vi "p72MomenInv.vi"(1 "Array 3":dbl[][](array[numeric])) -> (0 "appended array":dbl[](array[numeric]))   [LabVIEW 2013]
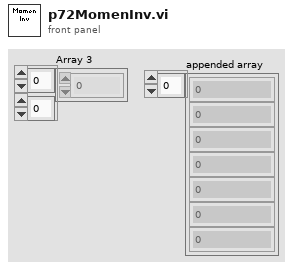
[diagram p1: front panel]
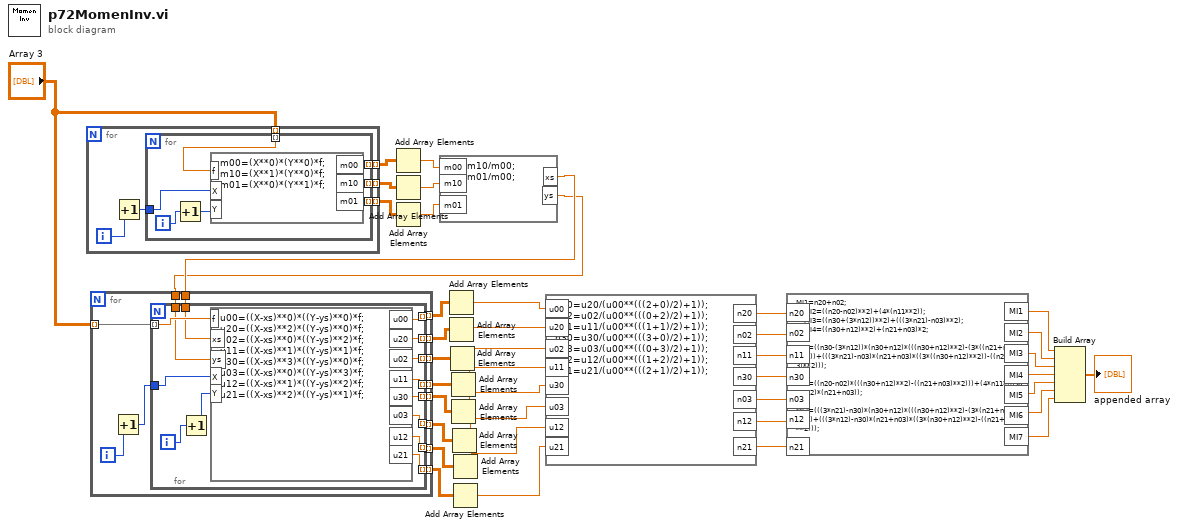
[diagram p0: block diagram]
diagram:
  n1 = for {
    tunnel: "Array 3" -> [w45] mode=indexing
    tunnel: [w43] -> w40 mode=indexing
    tunnel: [w42] -> w39 mode=indexing
    tunnel: [w41] -> w38 mode=indexing
    i -> [w46]
    n2 = Increment(x=w46) -> (x+1=w44:i32)
    n3 = for {
      tunnel: w45 -> [w53] mode=indexing
      tunnel: w44 -> [w52]
      tunnel: [w49] -> w43 mode=indexing
      tunnel: [w48] -> w42 mode=indexing
      tunnel: [w47] -> w41 mode=indexing
      i -> [w51]
      n4 = Increment(x=w51) -> (x+1=w50:i32)
      n5 = formula code="m00=(X**0)*(Y**0)*f;\nm10=(X**1)*(Y**0)*f;\nm01=(X**0)*(Y**1)*f;"("X"=w52, "Y"=w50, "f"=w53) -> ("m00"=w49:dbl, "m10"=w48:dbl, "m01"=w47:dbl)
    }
  }
  n6 = Add Array Elements(numeric array=w40) -> (sum=w37:dbl)
  n7 = Add Array Elements(numeric array=w39) -> (sum=w36:dbl)
  n8 = Add Array Elements(numeric array=w38) -> (sum=w35:dbl)
  n9 = formula code="xs=m10/m00;\nys=m01/m00;"("m00"=w37, "m10"=w36, "m01"=w35) -> ("xs"=w34:dbl, "ys"=w33:dbl)
  n10 = for {
    tunnel: "Array 3" -> [w66] mode=indexing
    tunnel: w34 -> [w65]
    tunnel: w33 -> [w64]
    tunnel: [w61] -> w32 mode=indexing
    tunnel: [w60] -> w31 mode=indexing
    tunnel: [w59] -> w30 mode=indexing
    tunnel: [w58] -> w29 mode=indexing
    tunnel: [w57] -> w28 mode=indexing
    tunnel: [w56] -> w27 mode=indexing
    tunnel: [w55] -> w26 mode=indexing
    tunnel: [w54] -> w25 mode=indexing
    i -> [w63]
    n11 = Increment(x=w63) -> (x+1=w62:i32)
    n12 = for {
      tunnel: w66 -> [w80] mode=indexing
      tunnel: w65 -> [w79]
      tunnel: w64 -> [w78]
      tunnel: w62 -> [w77]
      tunnel: [w74] -> w61 mode=indexing
      tunnel: [w73] -> w60 mode=indexing
      tunnel: [w72] -> w59 mode=indexing
      tunnel: [w71] -> w58 mode=indexing
      tunnel: [w70] -> w57 mode=indexing
      tunnel: [w69] -> w56 mode=indexing
      tunnel: [w68] -> w55 mode=indexing
      tunnel: [w67] -> w54 mode=indexing
      i -> [w76]
      n13 = Increment(x=w76) -> (x+1=w75:i32)
      n14 = formula code="u00=((X-xs)**0)*((Y-ys)**0)*f;\nu20=((X-xs)**2)*((Y-ys)**0)*f;\nu02=((X-xs)**0)*((Y-ys)**2)*f;\nu11=((X-xs)**1)*((Y-ys)**1)*f;\nu30=((X-xs)**3)*((Y-ys)**0)*f;\nu03=((X-xs)**0)*((Y-ys)**3)*f;\nu12=((X-xs)**1)*((Y-ys)**2)*f;\nu21=((X-xs)**2)*((Y-ys)**1)*f;"("f"=w80, "xs"=w79, "ys"=w78, "X"=w77, "Y"=w75) -> ("u00"=w74:dbl, "u20"=w73:dbl, "u02"=w72:dbl, "u11"=w71:dbl, "u30"=w70:dbl, "u03"=w69:dbl, "u12"=w68:dbl, "u21"=w67:dbl)
    }
  }
  n15 = Add Array Elements(numeric array=w32) -> (sum=w24:dbl)
  n16 = Add Array Elements(numeric array=w31) -> (sum=w23:dbl)
  n17 = Add Array Elements(numeric array=w30) -> (sum=w22:dbl)
  n18 = Add Array Elements(numeric array=w29) -> (sum=w21:dbl)
  n19 = Add Array Elements(numeric array=w28) -> (sum=w20:dbl)
  n20 = Add Array Elements(numeric array=w27) -> (sum=w19:dbl)
  n21 = Add Array Elements(numeric array=w26) -> (sum=w18:dbl)
  n22 = Add Array Elements(numeric array=w25) -> (sum=w17:dbl)
  n23 = formula code="n20=u20/(u00**(((2+0)/2)+1));\nn02=u02/(u00**(((0+2)/2)+1));\nn11=u11/(u00**(((1+1)/2)+1));\nn30=u30/(u00**(((3+0)/2)+1));\nn03=u03/(u00**(((0+3)/2)+1));\nn12=u12/(u00**(((1+2)/2)+1));\nn21=u21/(u00**(((2+1)/2)+1));"("u00"=w24, "u20"=w23, "u02"=w22, "u11"=w21, "u30"=w20, "u03"=w19, "u12"=w18, "u21"=w17) -> ("n20"=w16:dbl, "n02"=w15:dbl, "n11"=w14:dbl, "n30"=w13:dbl, "n03"=w12:dbl, "n12"=w11:dbl, "n21"=w10:dbl)
  n24 = formula code="MI1=n20+n02;\n    MI2=((n20-n02)**2)+(4*(n11**2));\n    MI3=((n30+(3*n12))**2)+(((3*n21)-n03)**2);\n    MI4=((n30+n12)**2)+(n21+n03)*2;\n    MI5=((n30-(3*n12))*(n30+n12)*(((n30+n12)**2)-(3*((n21+n03)**2))))+(((3*n21)-n03)*(n21+n03)*((3*((n30+n12)**2))-((n21+n03)**2)));\n    MI6=((n20-n02)*(((n30+n12)**2)-((n21+n03)**2)))+(4*n11*(n30+n12)*(n21+n03));\n    MI7=(((3*n21)-n30)*(n30+n12)*(((n30+n12)**2)-(3*(n21+n03)**2)))+(((3*n12)-n30)*(n21+n03)*((3*(n30+n12)**2)-((n21+n03)**2)));"("n20"=w16, "n02"=w15, "n11"=w14, "n30"=w13, "n03"=w12, "n12"=w11, "n21"=w10) -> ("MI1"=w9:dbl, "MI2"=w8:dbl, "MI3"=w7:dbl, "MI4"=w6:dbl, "MI5"=w5:dbl, "MI6"=w4:dbl, "MI7"=w3:dbl)
  n25 = Build Array(w9, w8, w7, w6, w5, w4, w3) -> (→"appended array":dbl[])
